vi "Piezo Message Loop.vi"(8 "error in (no error)":errorcluster, 11 "Message Queues":T1) -> (0 "error out":errorcluster)   [LabVIEW 2017, in "Piezo Controller.lvlib"]
uses:
  Piezo Controller.lvlib
  Vibratome/Message Queues.ctl
  Support VIs/Message Queue/Message.ctl
  FPGA Refs.ctl
  <instrlib>/_niInstr/FIFO Register Bus/v1/Host/niInstr FIFO Register Bus v1 Host.lvclass
  <instrlib>/_niInstr/Instruction Framework/v1/Host/Instruction Framework Context/niInstr Instruction Framework Context v1 Host.lvclass
  <vilib>/Utility/error.llb/Error Cluster From Error Code.vi
  Support VIs/Message Queue/Enqueue Message (Single).vi
  <vilib>/ErrorRing/Error Ring.xnode
  Support VIs/Message Queue/Message Queue.lvlib
  Vibratome/Vibratome.lvlib
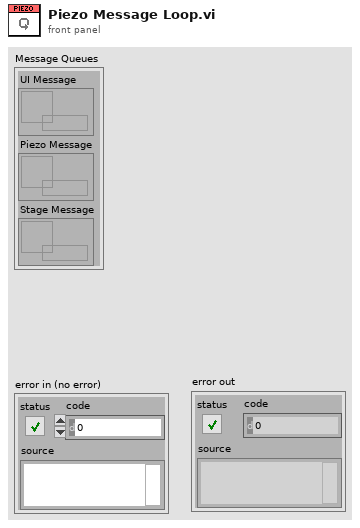
[diagram p1: front panel]
types:
  T1 = typedef "Vibratome.lvlib/Message Queues.ctl" = cluster{"UI Message":refnum<queue>, "Piezo Message":refnum<queue>, "Stage Message":refnum<queue>}
  T2 = typedef "Piezo Controller.lvlib/FPGA Refs.ctl" = cluster{"FPGA VI Reference":refnum<k20>, "Instruction Target":refnum<class "niInstr FIFO Register Bus v1 Host.lvclass">, "Context":refnum<class "niInstr Instruction Framework Context v1 Host.lvclass">}
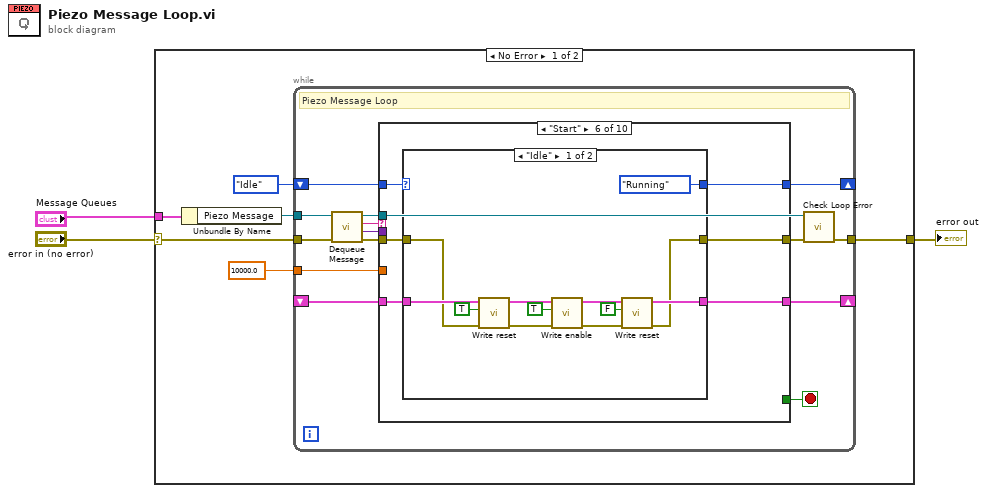
[diagram p0: block diagram]
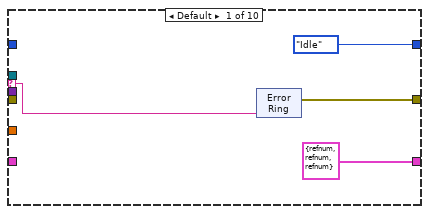
[diagram p2: hidden frame]
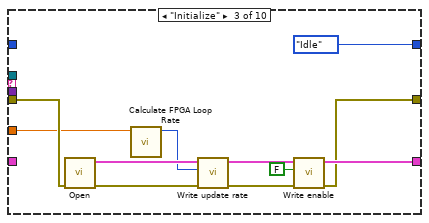
[diagram p4: hidden frame]
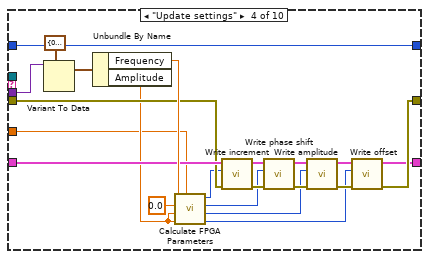
[diagram p5: hidden frame]
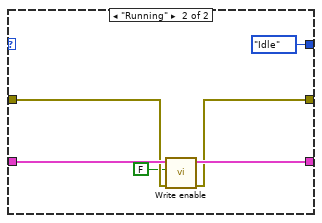
[diagram p9: hidden frame]
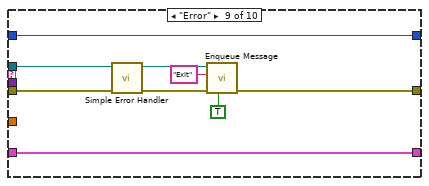
[diagram p11: hidden frame]
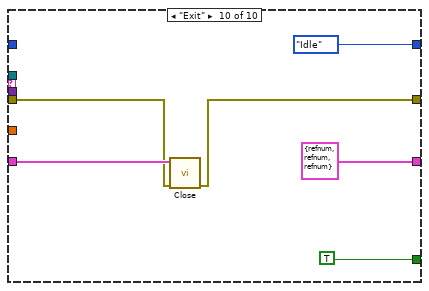
[diagram p12: hidden frame]
diagram:
  n1 = case shown="No Error" "error in (no error)" {
    selector: "error in (no error)" -> [w8 w127]
    tunnel: "Message Queues" -> [w9 _]
    tunnel: [w6 w127] -> w1
    frame No Error {
      n2 = Unbundle By Name(w9) -> ("Piezo Message"=w7:refnum<queue>)
      n3 = while {
        tunnel: w8 -> [w23]
        tunnel: w7 -> [w17]
        tunnel: [w16] -> w6
        shift-right: [w14] -> _
        shift-left: enum16{"Idle", "Running"}."Idle" -> [w15]
        shift-right: [w13] -> _
        shift-left: _ -> [w12]
        tunnel: 10000.0 ("Loop Frequency (Hz)") -> [w10]
        stop <- w18 stop-if-true
        # "Piezo Message Loop"
        n4 = call "Dequeue Message.vi"("error in (no error)"=w23, "Message Queue in"=w17) -> ("error out"=w21:errorcluster, "Data"=w11:variant, "State"=w22:string, "Message Queue out"=w20:refnum<queue>)  [unwired: 6 in]
        n5 = case shown="\"Start\"" w22 {
          selector: w22 -> [w26 _ _ _ _ _ _ _ _ _]
          tunnel: w20 -> [_ _ _ _ _ _ _ _ w115 _]
          tunnel: w21 -> [_ w37 w47 w59 w73 w76 w97 w112 w120 w123]
          tunnel: [w27 w37 w39 w55 w73 w77 w98 w112 w116 w122] -> w19
          tunnel: [_ _ _ _ _ _ _ _ _ TRUE] -> w18
          tunnel: w15 -> [_ w36 _ w70 w72 w79 w100 w111 w119 _]
          tunnel: [enum16{"Idle", "Running"}."Idle" w36 enum16{"Idle", "Running"}."Idle" w70 w72 w78 w99 w111 w119 enum16{"Idle", "Running"}."Idle"] -> w14
          tunnel: [T2 {"FPGA VI Reference"=refnum, "Instruction Target"=refnum, "Context"=refnum} ("FPGA Refs") w35 w41 w53 w71 w75 w95 w110 w118 T2 {"FPGA VI Reference"=refnum, "Instruction Target"=refnum, "Context"=refnum} ("FPGA Refs")] -> w13
          tunnel: w12 -> [_ w35 _ w60 w71 w74 w96 w110 w118 w124]
          tunnel: w11 -> [_ _ _ w69 _ _ _ _ _ _]
          tunnel: w10 -> [_ _ w43 w49 _ _ _ _ _ _]
          frame Default {
            n6 = xnode "Error Ring"("parameter 0"=w26) -> ("error out"=w27:errorcluster)
          }
          frame "--- SETUP ---" {
          }
          frame "Initialize" {
            n7 = call "Open.vi"("error in (no error)"=w47) -> ("error out"=w46:errorcluster, "FPGA Refs"=w45:T2)  [unwired: 9 in]
            n8 = call "Calculate FPGA Loop Rate.vi"("Loop Frequency (Hz)"=w43) -> ("Loop  Rate (ticks)"=w42:u32)  [unwired: 10 in]
            n9 = call "Write update rate.vi"("error in (no error)"=w46, "Loop  Rate (ticks)"=w42, "FPGA Refs in"=w45) -> ("error out"=w40:errorcluster, "FPGA Refs out"=w44:T2)  [unwired: 7 in]
            n10 = call "Write enable.vi"("error in (no error)"=w40, "Enable"=FALSE, "FPGA Refs in"=w44) -> ("error out"=w39:errorcluster, "FPGA Refs out"=w41:T2)  [unwired: 7 in]
          }
          frame "Update settings" {
            n11 = Variant To Data(type=cluster{"Amplitude":dbl, "Frequency":dbl} {"Amplitude"=0.0, "Frequency"=0.0} ("Oscillator Settings"), Variant=w69) -> (data=w67:cluster{"Amplitude":dbl, "Frequency":dbl})  [unwired: 1 in, 1 out]
            n12 = Unbundle By Name(w67) -> ("Frequency"=w66:dbl, "Amplitude"=w50:dbl)
            n13 = call "Calculate FPGA Parameters.vi"("Loop Rate (Hz)"=w49, "Signal Offset (V)"=w50, "Signal Amplitude (V)"=w50, "Phase Shift (Deg)"=0.0, "DDS Signal Frequency (Hz)"=w66) -> ("AO Offset"=w51:i16, "AO Amplitude"=w56:u16, "Phase Shift"=w57:u32, "Accumulator Increment"=w58:u32)  [unwired: 2 in, 1 out]
            n14 = call "Write increment.vi"("error in (no error)"=w59, "Increment"=w58, "FPGA Refs in"=w60) -> ("error out"=w64:errorcluster, "FPGA Refs out"=w61:T2)  [unwired: 7 in]
            n15 = call "Write phase shift.vi"("error in (no error)"=w64, "Phase shift"=w57, "FPGA Refs in"=w61) -> ("error out"=w63:errorcluster, "FPGA Refs out"=w62:T2)  [unwired: 7 in]
            n16 = call "Write amplitude.vi"("error in (no error)"=w63, "Amplitude"=w56, "FPGA Refs in"=w62) -> ("error out"=w54:errorcluster, "FPGA Refs out"=w52:T2)  [unwired: 7 in]
            n17 = call "Write offset.vi"("error in (no error)"=w54, "Offset"=w51, "FPGA Refs in"=w52) -> ("error out"=w55:errorcluster, "FPGA Refs out"=w53:T2)  [unwired: 7 in]
          }
          frame "--- OPS ---" {
          }
          frame "Start" {
            n18 = case shown="\"Idle\"" w79 {
              selector: w79 -> [_ w94]
              tunnel: [enum16{"Idle", "Running"}."Running" w94] -> w78
              tunnel: [w80 w93] -> w77
              tunnel: w76 -> [w85 w93]
              tunnel: [w83 w92] -> w75
              tunnel: w74 -> [w90 w92]
              frame "Idle" {
                n19 = call "Write reset.vi"("error in (no error)"=w85, "Enable"=TRUE, "FPGA Refs in"=w90) -> ("error out"=w84:errorcluster, "FPGA Refs out"=w87:T2)  [unwired: 7 in]
                n20 = call "Write enable.vi"("error in (no error)"=w84, "Enable"=TRUE, "FPGA Refs in"=w87) -> ("error out"=w81:errorcluster, "FPGA Refs out"=w89:T2)  [unwired: 7 in]
                n21 = call "Write reset.vi"("error in (no error)"=w81, "Enable"=FALSE, "FPGA Refs in"=w89) -> ("error out"=w80:errorcluster, "FPGA Refs out"=w83:T2)  [unwired: 7 in]
              }
              frame "Running" {
              }
            }
          }
          frame "Stop" {
            n22 = case shown="\"Idle\"" w100 {
              selector: w100 -> [w103 _]
              tunnel: [w103 enum16{"Idle", "Running"}."Idle"] -> w99
              tunnel: [w102 w105] -> w98
              tunnel: w97 -> [w102 w106]
              tunnel: w96 -> [w101 w108]
              tunnel: [w101 w107] -> w95
              frame "Idle" {
              }
              frame "Running" {
                n23 = call "Write enable.vi"("error in (no error)"=w106, "Enable"=FALSE, "FPGA Refs in"=w108) -> ("error out"=w105:errorcluster, "FPGA Refs out"=w107:T2)  [unwired: 7 in]
              }
            }
          }
          frame "--- MISC ---" {
          }
          frame "Error" {
            n24 = call <vilib>:"Simple Error Handler.vi"("error in (no error)"=w120) -> ("error out"=w117:errorcluster)  [unwired: 4 in, 4 out]
            n25 = call-poly "Enqueue Message.vi"("High Priority?"=TRUE, "error in (no error)"=w117, "State"="Exit", "Message Queue in"=w115) -> ("error out"=w116:errorcluster)  [unwired: 6 in, 1 out]
          }
          frame "Exit" {
            n26 = call "Close.vi"("error in (no error)"=w123, "FPGA Refs"=w124) -> ("error out"=w122:errorcluster)  [unwired: 9 in]
          }
        }
        n27 = call "Check Loop Error.vi"("error in (no error)"=w19, "Message Queue in"=w20) -> ("error out"=w16:errorcluster)  [unwired: 7 in, 2 out]
      }
    }
    frame Error {
    }
  }
  "error out" <- w1
